vi "table_get_subtable_item.vi"(7 "subtables":string[](array[string]), 8 "error in (no error)":errorcluster, 10 "subkeys":string[](array[string]), 11 "Table in":refnum<class "Table.lvclass">) -> (0 "error out":errorcluster, 1 "item (value)":refnum<class "Item.lvclass">, 2 "found?":bool, 3 "Table out":refnum<class "Table.lvclass">)   [LabVIEW 2020, in "toml.lvclass"]
uses:
  toml.lvclass
  Item/Item.lvclass
  Table/Table.lvclass
  toml.lvclass/toml.ctl
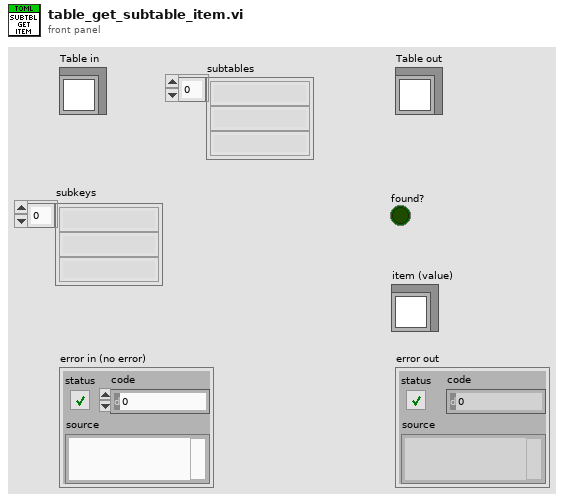
[diagram p1: front panel]
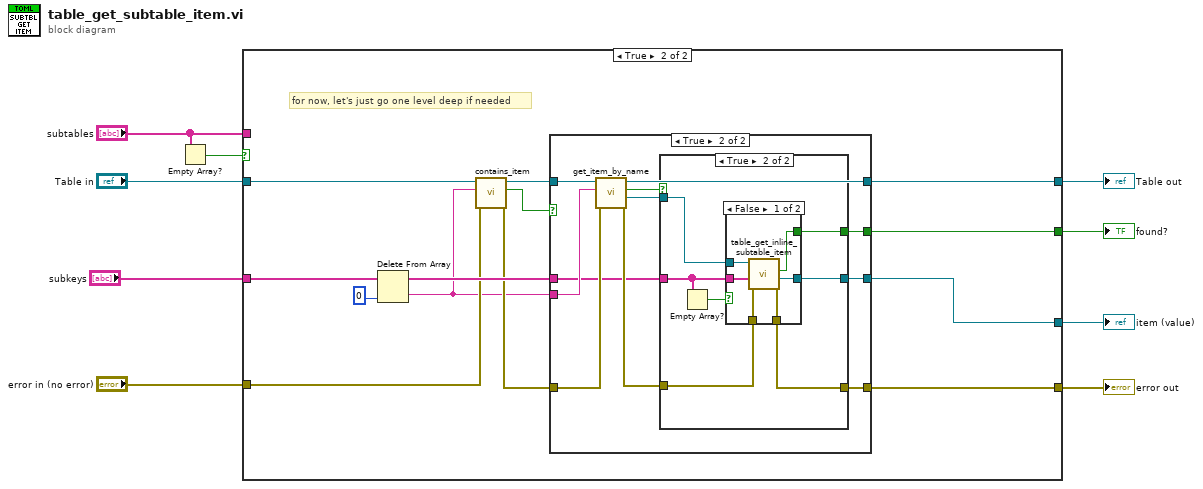
[diagram p0: block diagram]
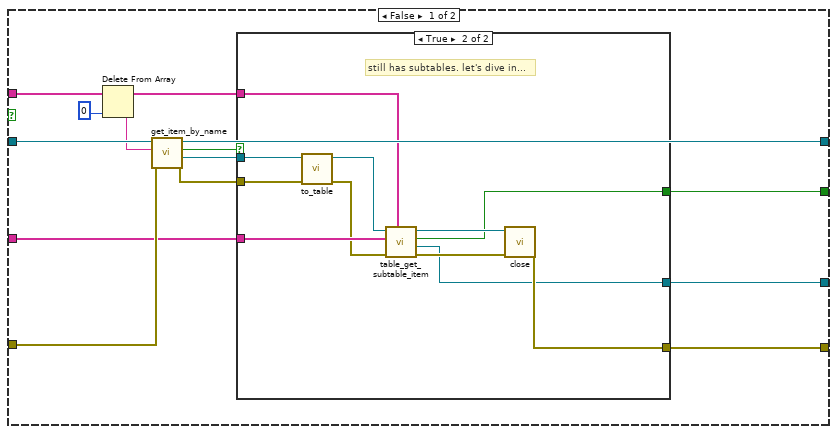
[diagram p2: hidden frame]
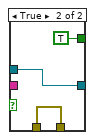
[diagram p6: hidden frame]
diagram:
  n1 = Empty Array?(array="subtables") -> (empty?=w4:bool)
  n2 = case shown="True" w4 {
    tunnel: [w14 w42] -> w9
    tunnel: "subkeys" -> [w12 w45]
    tunnel: [w17 w44] -> w7
    tunnel: "Table in" -> [w20 w40]
    tunnel: "error in (no error)" -> [w19 w38]
    tunnel: "subtables" -> [w23 _]
    tunnel: [w13 w48] -> w2
    tunnel: [w11 w47] -> w1
    frame False {
      n3 = Delete From Array(array=w23, index=0) -> (deleted portion=w15:string, array with subset deleted=w21:string[])  [unwired: 1 in]
      n4 = call "get_item_by_name.vi"("error in (no error)"=w19, "item_name"=w15, "Table in"=w20) -> ("error out"=w16:errorcluster, "Item"=w18:refnum<class "Item.lvclass">, "found?"=w10:bool, "Table out"=w17:refnum<class "Table.lvclass">)  [unwired: 4 in, 1 out]
      n5 = case shown="True" w10 {
        tunnel: w21 -> [_ w35]
        tunnel: w18 -> [_ w34]
        tunnel: w16 -> [w24 w33]
        tunnel: [w24 w30] -> w14
        tunnel: [_ w29] -> w13
        tunnel: w12 -> [_ w28]
        tunnel: [_ w25] -> w11
        frame False {
        }
        frame True {
          # "still has subtables. let's dive in..."
          n6 = call "to_table.vi"("error in (no error)"=w33, "Item in"=w34) -> ("error out"=w27:errorcluster, "Table"=w26:refnum<class "Table.lvclass">)  [unwired: 8 in]
          n7 = call "table_get_subtable_item.vi"("subtables"=w35, "error in (no error)"=w27, "subkeys"=w28, "Table in"=w26) -> ("error out"=w31:errorcluster, "item (value)"=w29:refnum<class "Item.lvclass">, "found?"=w25:bool, "Table out"=w32:refnum<class "Table.lvclass">)  [unwired: 4 in]
          n8 = call "close.vi"("error in (no error)"=w31, "Table in"=w32) -> ("error out"=w30:errorcluster)  [unwired: 9 in]
        }
      }
    }
    frame True {
      # "for now, let's just go one level deep if needed"
      n9 = Delete From Array(array=w45, index=0) -> (deleted portion=w36:string, array with subset deleted=w43:string[])  [unwired: 1 in]
      n10 = call "contains_item.vi"("error in (no error)"=w38, "item_name"=w36, "Table in"=w40) -> ("error out"=w39:errorcluster, "contains_item"=w37:bool, "Table out"=w41:refnum<class "Table.lvclass">)  [unwired: 6 in]
      n11 = case shown="True" w37 {
        tunnel: [_ w61] -> w48
        tunnel: [_ w60] -> w47
        tunnel: w36 -> [_ w59]
        tunnel: [w49 w58] -> w44
        tunnel: w43 -> [_ w52]
        tunnel: [w50 w55] -> w42
        tunnel: w41 -> [w49 w54]
        tunnel: w39 -> [w50 w53]
        frame False {
        }
        frame True {
          n12 = call "get_item_by_name.vi"("error in (no error)"=w53, "item_name"=w59, "Table in"=w54) -> ("error out"=w56:errorcluster, "Item"=w57:refnum<class "Item.lvclass">, "found?"=w51:bool, "Table out"=w58:refnum<class "Table.lvclass">)  [unwired: 4 in, 1 out]
          n13 = case shown="True" w51 {
            tunnel: [_ w69] -> w61
            tunnel: [_ w68] -> w60
            tunnel: w57 -> [_ w67]
            tunnel: w56 -> [w62 w66]
            tunnel: [w62 w65] -> w55
            tunnel: w52 -> [_ w64]
            frame False {
            }
            frame True {
              n14 = Empty Array?(array=w64) -> (empty?=w63:bool)
              n15 = case shown="False" w63 {
                tunnel: [w75 w78] -> w69
                tunnel: [w74 TRUE ("contains_item")] -> w68
                tunnel: w67 -> [w73 w78]
                tunnel: w66 -> [w72 w76]
                tunnel: [w71 w76] -> w65
                tunnel: w64 -> [w70 _]
                frame False {
                  n16 = call "table_get_inline_subtable_item.vi"("error in (no error)"=w72, "subkeys"=w70, "Item in"=w73) -> ("error out"=w71:errorcluster, "Item"=w75:refnum<class "Item.lvclass">, "contains_item"=w74:bool)  [unwired: 6 in]
                }
                frame True {
                }
              }
            }
          }
        }
      }
    }
  }
  "error out" <- w9
  "item (value)" <- w2
  "Table out" <- w7
  "found?" <- w1
